vi "Error if not valid Test Suite.vi"(8 "error in (no error)":errorcluster, 11 "Test Suite":refnum<class "Test Suite.lvclass">) -> (0 "error out":errorcluster)   [LabVIEW 2013, in "JUnit XML.lvlib" / "Test Suites.lvclass"]
doc: "Creates an error if <B>Test Suite</B> does not have a valid <B>Package</B> or <B>Id</B>."
uses:
  Test Suites.lvclass
  Test Suite/Test Suite.lvclass
  Test Suite/Test Suite.lvclass/Test Suite.ctl
  Test Suite/Read Package.vi
  Test Suite/Read Id.vi
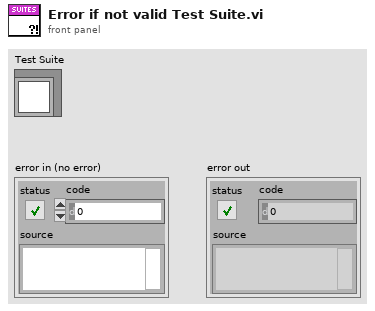
[diagram p1: front panel]
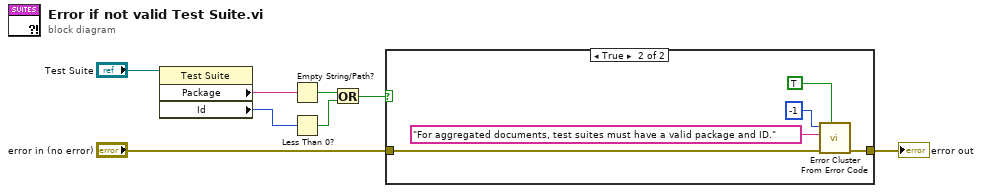
[diagram p0: block diagram]
diagram:
  n1 = property class="Test Suite"(reference="Test Suite") -> ("Package"=w7:string, "Id"=w6:i32)  [unwired: 1 in, 2 out]
  n2 = Empty String/Path?(string/path=w7) -> (empty?=w5:bool)
  n3 = Less Than 0?(x=w6) -> (x < 0?=w4:bool)
  n4 = Or(x=w5, y=w4) -> (x .or. y?=w3:bool)
  n5 = case shown="True" w3 {
    tunnel: "error in (no error)" -> [w9 w14]
    tunnel: [w9 w13] -> w1
    frame False {
    }
    frame True {
      n6 = call <vilib>:"Error Cluster From Error Code.vi"("show call chain? (False)"=TRUE, "error in (no error)"=w14, "error message (\"\")"="For aggregated documents, test suites must have a valid package and ID." ("error message (\"\")"), "error code (0)"=-1) -> ("error out"=w13:errorcluster)  [unwired: 5 in]
    }
  }
  "error out" <- w1
